vi "FTW-Message-Receive.vi"(0 "FTW Incoming Message":refnum<class "FTW-Message.lvclass">, 11 "error in":errorcluster) -> (4 "FTW Incoming Message out":refnum<class "FTW-Message.lvclass">, 6 "Message":string, 15 "error out":errorcluster)   [LabVIEW 2013, in "FTW-Message.lvclass"]
uses:
  FTW-Message.lvclass
  FTW-Message.lvclass/FTW-Message.ctl
panel:
  # "Inputs"
  # "Outputs"
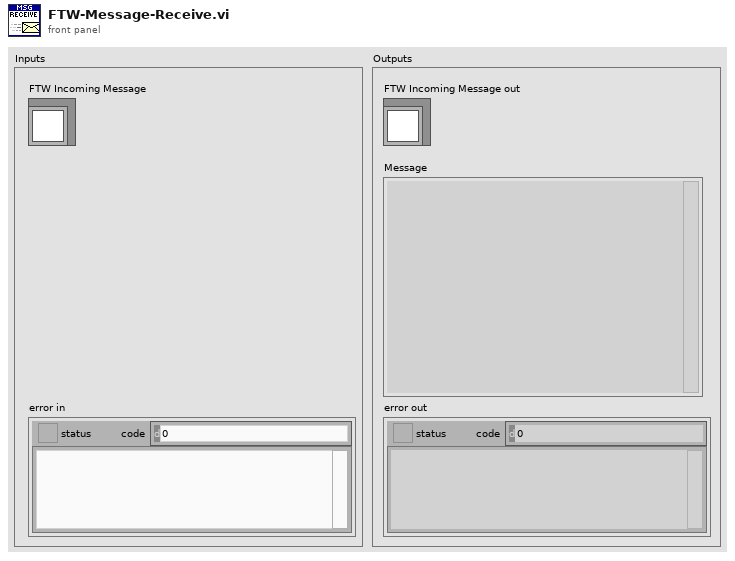
[diagram p1: front panel]
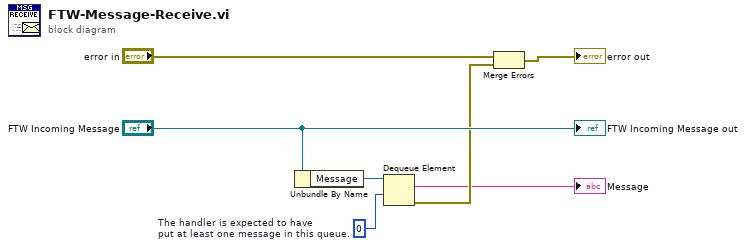
[diagram p0: block diagram]
diagram:
  w1 = 0  # The handler is expected to have put at least one message in this queue.
  n1 = Unbundle By Name("FTW Incoming Message") -> ("Message"=w6:refnum<queue>)
  n2 = Dequeue Element(queue=w6, timeout in ms (-1)=w1) -> (element=→"Message":string, error out=w3:errorcluster)  [unwired: 1 in, 2 out]
  n3 = Merge Errors("error in", w3) -> (→"error out":errorcluster)
  "FTW Incoming Message out" <- "FTW Incoming Message"
